vi "GetRightSideInformation.vi"(8 "error in (no error)":errorcluster, 10 "Left position":T1, 11 "EAN-13 in":refnum<class "EAN-13.lvclass">) -> (0 "error out":errorcluster, 2 "Right text position":T1, 3 "EAN-13 out":refnum<class "EAN-13.lvclass">)   [LabVIEW 2013, in "BarCodes.lvlib" / "EAN-13.lvclass"]
uses:
  EAN-13.lvclass
  BarCode/TextPosition.ctl
  BarCodes.lvlib
  BarCode/BarCode.lvclass
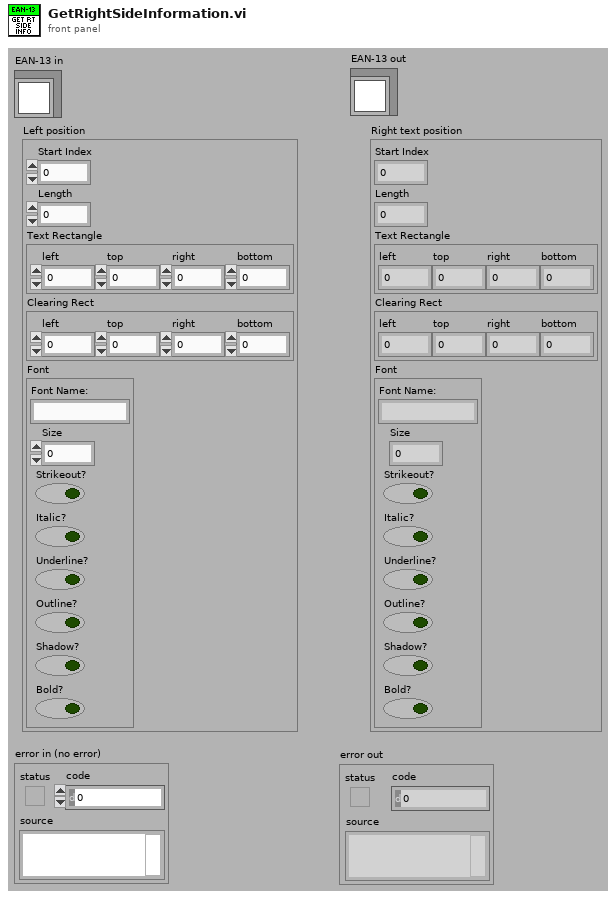
[diagram p1: front panel]
types:
  T1 = typedef "BarCodes.lvlib/BarCode.lvclass/TextPosition.ctl" = cluster{"Start Index":u8, "Length":u8, "Text Rectangle":cluster{"left":i16, "top":i16, "right":i16, "bottom":i16}, "Clearing Rect":cluster{"left":i16, "top":i16, "right":i16, "bottom":i16}, "Font":cluster{"Font Name:":string, "Size":i16, "Strikeout?":bool, "Italic?":bool, "Underline?":bool, "Outline?":bool, "Shadow?":bool, "Bold?":bool}}
  T2 = cluster{"left":i16, "top":i16, "right":i16, "bottom":i16}
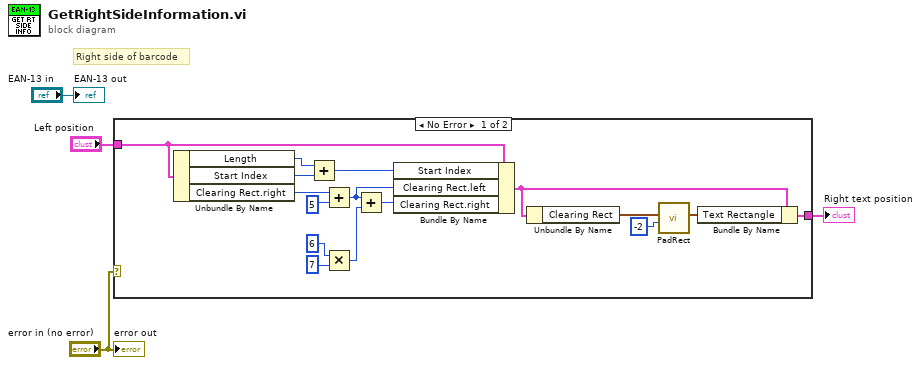
[diagram p0: block diagram]
diagram:
  # "Right side of barcode"
  n1 = case shown="No Error" "error in (no error)" {
    tunnel: "Left position" -> [w20 _]
    tunnel: [w19 _] -> w3
    frame No Error {
      n2 = Unbundle By Name(w20) -> ("Length"=w6:u8, "Start Index"=w7:u8, "Clearing Rect.right"=w8:i16)
      n3 = Add(x=w6, y=w7) -> (x+y=w5:u8)
      n4 = Add(x=w8, y=u8 5 ("End Index")) -> (x+y=w15:i16)
      n5 = Multiply(x=u8 6 ("End Index"), y=u8 7 ("End Index")) -> (x*y=w14:u8)
      n6 = Add(x=w15, y=w14) -> (x+y=w13:i16)
      n7 = Bundle By Name(cluster=w20, "Start Index"=w5, "Clearing Rect.left"=w15, "Clearing Rect.right"=w13) -> (w10:T1)
      n8 = Unbundle By Name(w10) -> ("Clearing Rect"=w12:T2)
      n9 = call "PadRect.vi"("Padding"=i8 -2, "Rectagle"=w12) -> ("Padded Rectangle"=w9:T2)  [unwired: 9 in]
      n10 = Bundle By Name(cluster=w10, "Text Rectangle"=w9) -> (w19:T1)
    }
    frame Error {
    }
  }
  "Right text position" <- w3
  "EAN-13 out" <- "EAN-13 in"
  "error out" <- "error in (no error)"
